vi "Add Quaternions.vi"(1 "quaternion 2":T1, 2 "quaternion 1":T1) -> (0 "sum":T1)   [LabVIEW 2017, in "NI_Kinematics.lvlib"]
doc: "Returns the sum of two quaternions."
uses:
  <vilib>/robotics/Kinematics/NI_Kinematics.lvlib
  <vilib>/robotics/Kinematics/Quaternion.ctl
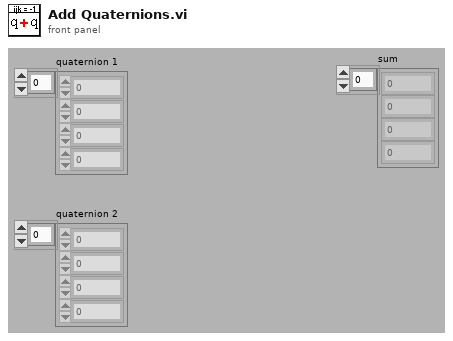
[diagram p1: front panel]
types:
  T1 = typedef "NI_Kinematics.lvlib/Quaternion.ctl" = dbl[]
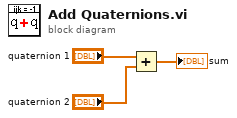
[diagram p0: block diagram]
diagram:
  n1 = Add(x="quaternion 1", y="quaternion 2") -> (x+y=→"sum":T1)
